vi "Open XL WorkBook.vi"(8 "error in":errorcluster, 9 "Workbook":T1, 10 "Workbooks":refnum<k7>, 11 "Excel._Application":refnum<k7>) -> (0 "error out":errorcluster, 1 "Sheets":refnum<k7>, 2 "Excel._Workbook":refnum<k7>, 3 "Excel.Workbooks":refnum<k7>)   [LabVIEW 2017]
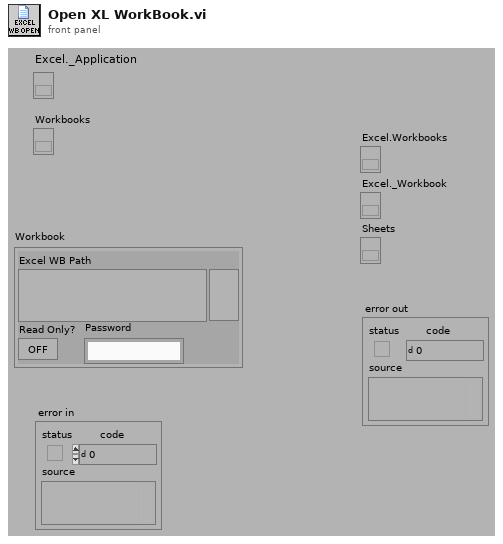
[diagram p1: front panel]
types:
  T1 = cluster{"Excel WB Path":path, "Read Only?":bool, "Password":string}
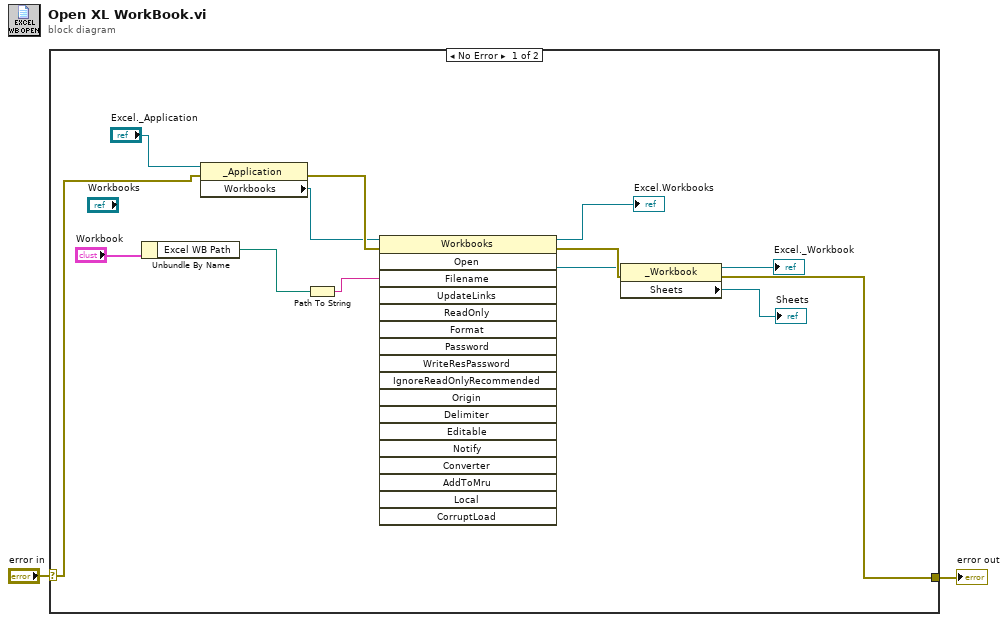
[diagram p0: block diagram]
diagram:
  n1 = case shown="No Error" "error in" {
    selector: "error in" -> [w6 w16]
    tunnel: [w15 w16] -> w1
    frame No Error {
      n2 = Unbundle By Name("Workbook") -> ("Excel WB Path"=w14:path)
      n3 = property class="_Application"(reference="Excel._Application", error in=w6) -> (error out=w5:errorcluster, "Workbooks"=w4:refnum<k7>)  [unwired: 1 out]
      n4 = Path To String(path=w14) -> (string=w11:string)
      n5 = invoke class="Workbooks" method="Open"(reference=w4, error in=w5, "Filename"=w11) -> (reference out=→"Excel.Workbooks":refnum<k7>, error out=w10:errorcluster, "Open"=w8:refnum<k7>)  [unwired: 15 in, 15 out]
      n6 = property class="_Workbook"(reference=w8, error in=w10) -> (reference out=→"Excel._Workbook":refnum<k7>, error out=w15:errorcluster, "Sheets"=→"Sheets":refnum<k7>)
    }
    frame Error {
    }
  }
  "error out" <- w1
